vi "836 Installer.vi"() -> ()   [LabVIEW 2014]
uses:
  <vilib>/Utility/sysdir.llb/System Directory Type.ctl
  <vilib>/zip/NI_Unzip.lvlib
panel:
  in  "OK Button":bool
  in  "User Lib":bool
  in  "Examples":bool
  out "836 Examples Install Directory":path
  out "LabVIEW user.lib Install Directory":path
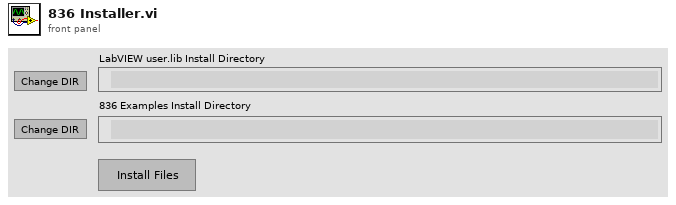
[diagram p1: front panel]
types:
  T1 = typedef "System Directory Type.ctl" = i32
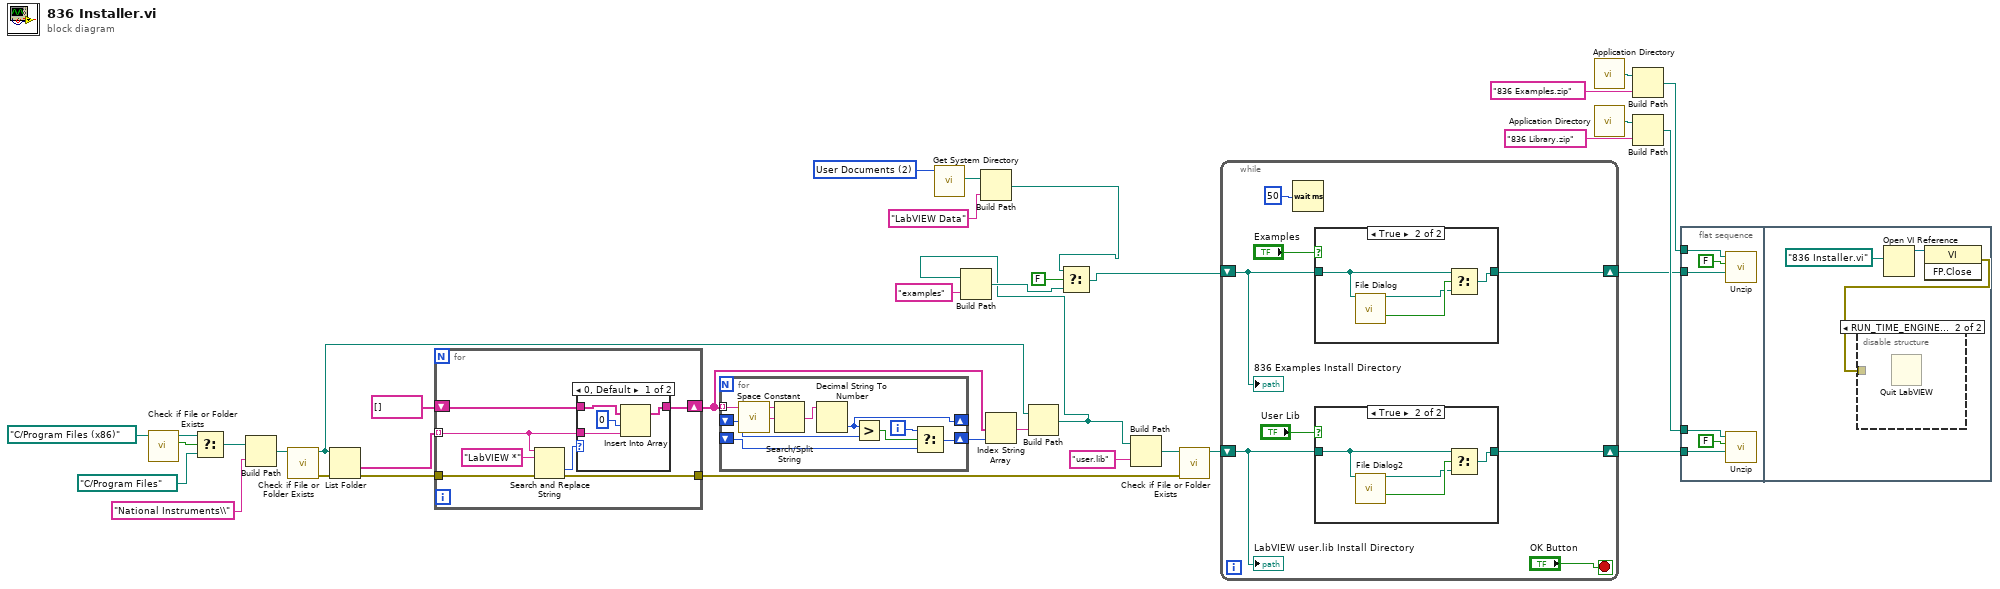
[diagram p0: block diagram]
diagram:
  w17 = T1 2 items=["User Home"=0, "User Desktop"=1, "User Documents"=2, "User Application Data"=3, "User Preferences"=4, "User Temporary"=5, "Public Documents"=6, "Public Application Data"=7, "Public Preferences"=8, "Public Cache"=13, "System Core Libraries"=9, "System Installed Libraries"=10, "Application Files"=11, "Boot Volume Root"=12] ("system directory type")
  n1 = call <vilib>:"Check if File or Folder Exists.vi"("path"=path "C:/Program Files (x86)") -> ("file or folder exists?"=w35:bool, "dup path"=w34:path)  [unwired: 8 in, 1 out]
  n2 = Select(t=w34, s=w35, f=path "C:/Program Files" ("path")) -> (s? t:f=w32:path)
  n3 = Build Path(base path=w32, name or relative path="National Instruments\\") -> (appended path=w30:path)
  n4 = call <vilib>:"Check if File or Folder Exists.vi"("path"=w30) -> ("error out"=w29:errorcluster, "dup path"=w4:path)  [unwired: 8 in, 1 out]
  n5 = List Folder(path=w4, error in=w29) -> (folder names=w26:string[], error out=w21:errorcluster)  [unwired: 2 in, 2 out]
  n6 = for {
    tunnel: w26 -> [w39] mode=indexing
    shift-right: [w42] -> w23
    shift-left: string[] [] ("folder names") -> [w43]
    tunnel: w21 -> [w38]
    tunnel: [w37] -> w20
    n7 = Search and Replace String(input string=w39, search string="LabVIEW *" ("pattern"), error in=w38) -> (offset past replacement=w40:i32, error out=w37:errorcluster)  [unwired: 5 in, 2 out]
    n8 = case shown="0, Default" w40 {
      tunnel: w43 -> [w47 w48]
      tunnel: [w46 w48] -> w42
      tunnel: w39 -> [w44 _]
      frame 0, Default {
        n9 = Insert Into Array(array=w47, index=0, new element=w44) -> (w46:string[])
      }
      frame -1 {
      }
    }
  }
  n10 = for {
    tunnel: w23 -> [w57] mode=indexing
    shift-right: [w54] -> _
    shift-left: _ -> [w53]
    shift-right: [w50] -> w24
    shift-left: _ -> [w49]
    i -> [w51]
    n11 = call <vilib>:"Space Constant.vi"() -> ("String"=w56:string)
    n12 = Search/Split String(string=w57, search string/char (-)=w56) -> (match + rest of string=w55:string)  [unwired: 1 in, 2 out]
    n13 = Decimal String To Number(string=w55) -> (number=w54:i32)  [unwired: 2 in, 1 out]
    n14 = Greater?(x=w54, y=w53) -> (0:w52:bool)
    n15 = Select(t=w51, s=w52, f=w49) -> (s? t:f=w50:i32)
  }
  n16 = call <vilib>:"Get System Directory.vi"("system directory type"=w17) -> ("system directory"=w15:path)  [unwired: 10 in]
  n17 = Build Path(base path=w15, name or relative path="LabVIEW Data") -> (appended path=w7:path)
  n18 = Index String Array(1:w24, 2:w23) -> (0:w22:string)  [unwired: 1 in]
  n19 = Build Path(base path=w4, name or relative path=w22) -> (appended path=w1:path)
  n20 = Build Path(base path=w1, name or relative path="examples") -> (appended path=w2:path)
  n21 = Select(t=w7, s=FALSE, f=w2) -> (s? t:f=w6:path)
  n22 = Build Path(base path=w1, name or relative path="user.lib") -> (appended path=w27:path)
  n23 = call <vilib>:"Check if File or Folder Exists.vi"("error in (no error)"=w20, "path"=w27) -> ("dup path"=w14:path)  [unwired: 7 in, 2 out]
  n24 = while {
    shift-right: [w63] -> w10
    shift-left: w6 -> [w65]
    shift-right: [w61] -> w13
    shift-left: w14 -> [w60]
    stop <- "OK Button" stop-if-true
    n25 = Wait (ms)(milliseconds to wait=u32 50) -> ()  [unwired: 1 out]
    n26 = case shown="True" "Examples" {
      tunnel: w65 -> [w71 w74]
      tunnel: [w71 w73] -> w63
      frame False {
      }
      frame True {
        n27 = call "File Dialog"("start path"=w74) -> ("selected path"=w72:path, "cancelled"=w75:bool)  [unwired: 11 in, 2 out]
        n28 = Select(t=w74, s=w75, f=w72) -> (s? t:f=w73:path)
      }
    }
    n29 = case shown="True" "User Lib" {
      tunnel: w60 -> [w66 w69]
      tunnel: [w66 w68] -> w61
      frame False {
      }
      frame True {
        n30 = call "File Dialog2"("start path"=w69) -> ("selected path"=w67:path, "cancelled"=w70:bool)  [unwired: 11 in, 2 out]
        n31 = Select(t=w69, s=w70, f=w67) -> (s? t:f=w68:path)
      }
    }
    "836 Examples Install Directory" <- w65
    "LabVIEW user.lib Install Directory" <- w60
  }
  n32 = call <vilib>:"Application Directory.vi"() -> ("Application Directory"=w8:path)
  n33 = call <vilib>:"Application Directory.vi"() -> ("Application Directory"=w9:path)
  n34 = Build Path(base path=w8, name or relative path="836 Examples.zip") -> (appended path=w12:path)
  n35 = Build Path(base path=w9, name or relative path="836 Library.zip") -> (appended path=w18:path)
  n36 = flat-sequence {
    tunnel: w18 -> [w81]
    tunnel: w13 -> [w79]
    tunnel: w12 -> [w78]
    tunnel: w10 -> [w77]
    frame #0 {
      n37 = call <vilib>:"Unzip.vi"("Target directory (same as Zip file if empty)"=w77, "Preview only?"=FALSE, "Zip file"=w78) -> ()  [unwired: 6 in, 3 out]
      n38 = call <vilib>:"Unzip.vi"("Target directory (same as Zip file if empty)"=w79, "Preview only?"=FALSE, "Zip file"=w81) -> ()  [unwired: 6 in, 3 out]
    }
    frame #1 {
      n39 = Open VI Reference(vi path=path "836 Installer.vi") -> (vi reference=w84:refnum<vi>)  [unwired: 5 in, 1 out]
      n40 = invoke class="VI" method="FP.Close"(reference=w84) -> (error out=w82:errorcluster)  [unwired: 2 in, 2 out]
      n41 = disable-structure shown="RUN_TIME_ENGINE==True" {
        disable-tunnel: w82 -> [_ _]
        frame condition #0 (active) {
        }
        frame condition #1 {
          n42 = Quit LabVIEW() -> ()  [unwired: 1 in]
        }
      }
    }
  }
